vi "S8300E_voltage_test_WIH.vi"() -> ()   [LabVIEW 2011]
uses:
  Instance          16 28Saved   KT300WR2_TP125B_PCBA .vi
  Instance          20 28Saved   KT300WR2_TP125B_PCBA .vi
panel:
  out "history log":string
  out "Log1":string
  out "DDR3 HL":string
  out "VRH":string[](array[string])
  out "VRL":string[](array[string])
  out "Measure Ai name":string
  out "VISA resource name out":refnum<visa-resource-name>
  out "SEARCHING Test Item":string[](array[string])
  out "SFCS_Network Ok?":bool=TRUE
  out "log_measured Voltage":string
  out "begin time":u32
  out "All Pass?":bool=TRUE
  out "Result(測試總結果)":bool
  out "Total TP":i32
  out "record(s)":T1(array[cluster])
  out "狀況":string
  out "Test Result (測試結果)":T2(array[cluster])
  # "S8300E  Voltage Test Points Check"
  # "2015-6-1"
  # "COM9  Baud 115200"
  # "Error Code\nP5V\nP3V3\nP1V8\nPVCCIO\nP1V0_PCH\nPVCCSA\nH-P1V5\nH-P0V75\nPVCCPLL\nP3V3_S0\nP1V05_PCH\nP1V5_PCH\nP1V8_PCH\n P3V3_PCH\nL-P1V5\nL-P0V75"
types:
  T1 = cluster{"TestPoint_Name":string, "Lower Limit Voltage":dbl, "High Limit Voltage":dbl, cluster{"Relay3 Name":string, "Relay3H/L":bool}[], "Measure Ai name":string}[]
  T2 = cluster{"Test Item":string, "SPEC MIN ":dbl, "SPEC MAX ":dbl, "Measured":dbl, bool}[]
  T3 = enum16{"open", "replace", "create", "open or create", "replace or create", "replace or create with confirmation"}
  T4 = cluster{"Test Item":string, "SPEC MIN V":dbl, "SPEC MAX V":dbl, "Measured V":dbl, bool}[]
  T5 = cluster{"Test Item":string, "SPEC MIN C":dbl, "SPEC MAX C":dbl, "Measured C":dbl, bool}
  T6 = cluster{"Test Item":string, "SPEC MIN C":dbl, "SPEC MAX C":dbl, "Measured C":dbl, bool}[]
  T7 = cluster{"TestPoint_Name":string, "Lower Limit Voltage":dbl, "High Limit Voltage":dbl, cluster{"Relay3 Name":string, "Relay3H/L":bool}[], "Measure Ai name":string}
  T8 = cluster{"Relay3 Name":string, "Relay3H/L":bool}[]
  T9 = cluster{"Test Item":string, "SPEC MIN ":dbl, "SPEC MAX ":dbl, "Measured":dbl, bool}
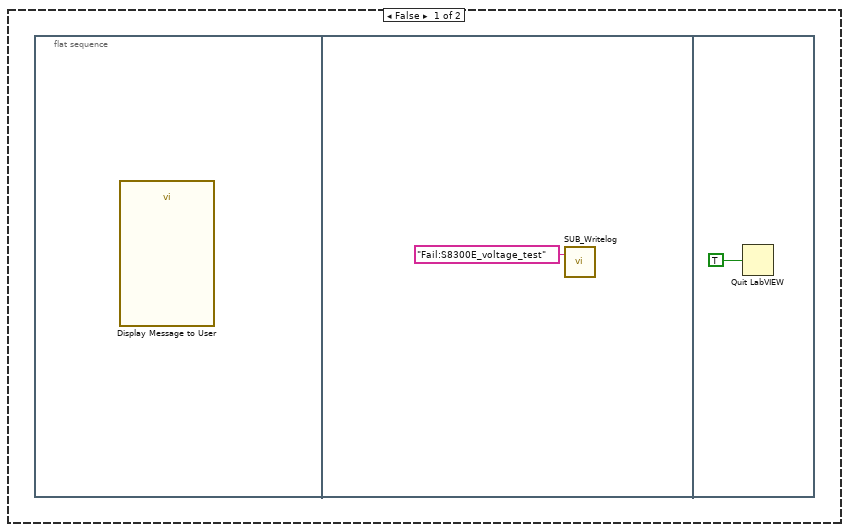
[diagram p2: hidden frame]
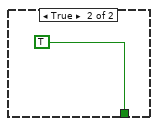
[diagram p5: hidden frame]
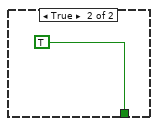
[diagram p8: hidden frame]
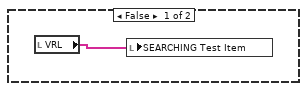
[diagram p9: hidden frame]
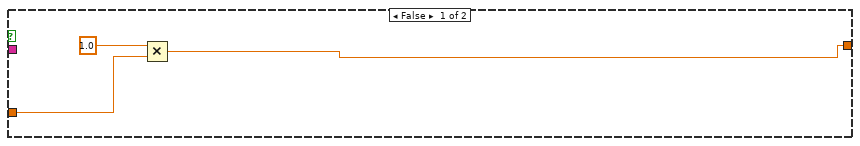
[diagram p12: hidden frame]
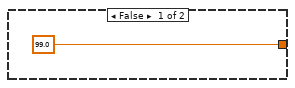
[diagram p13: hidden frame]
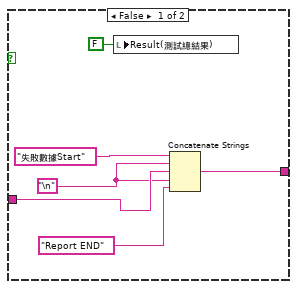
[diagram p15: hidden frame]
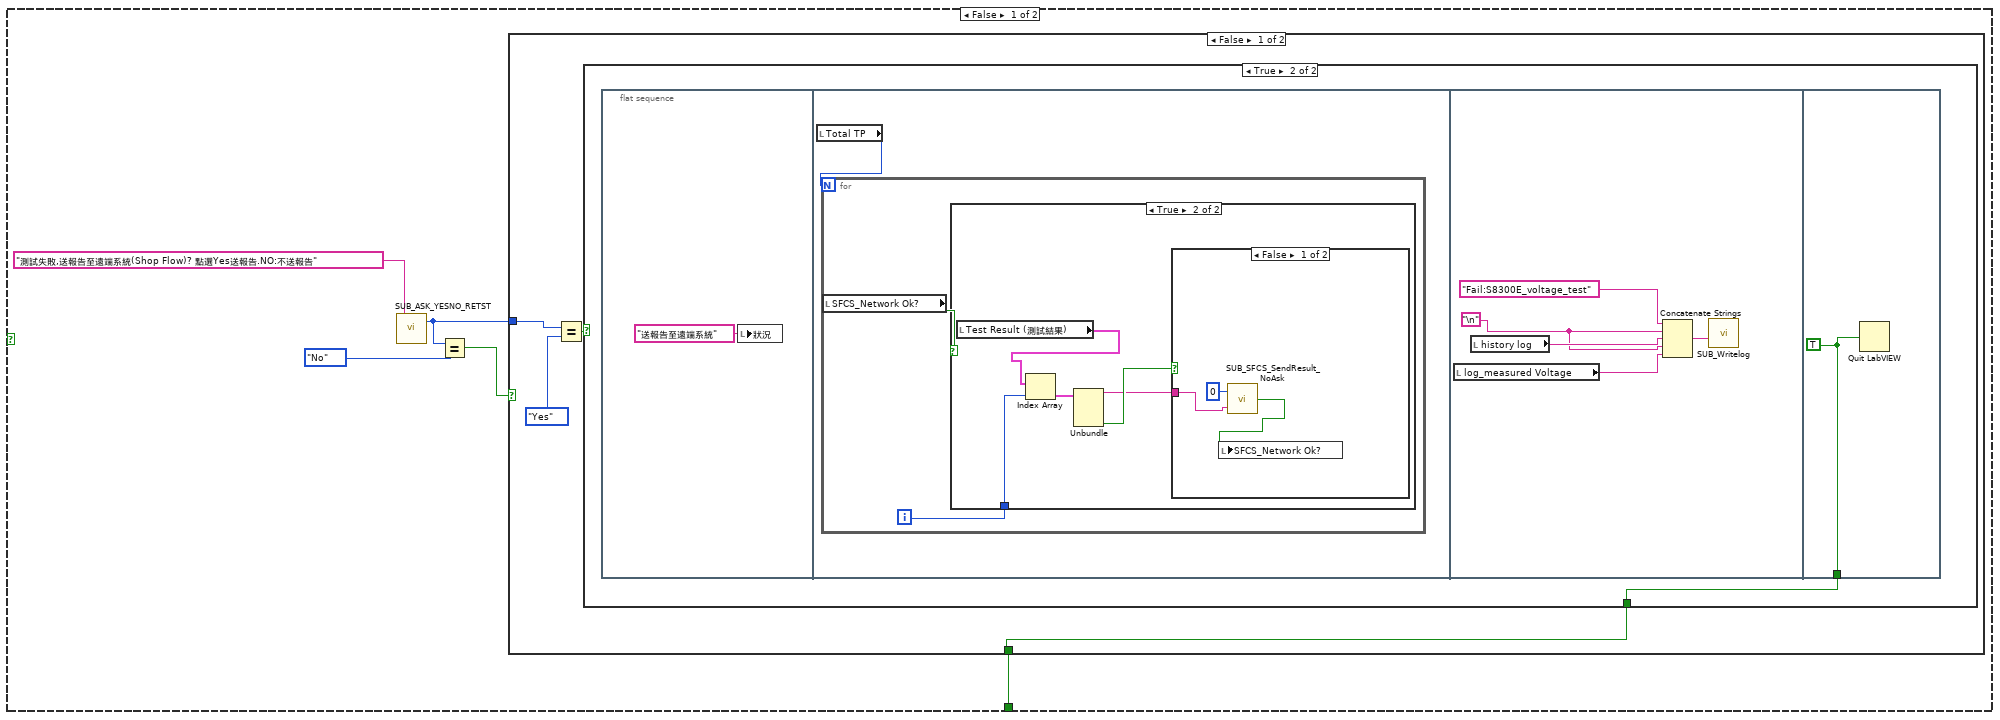
[diagram p16: hidden frame]
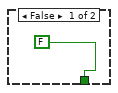
[diagram p17: hidden frame]
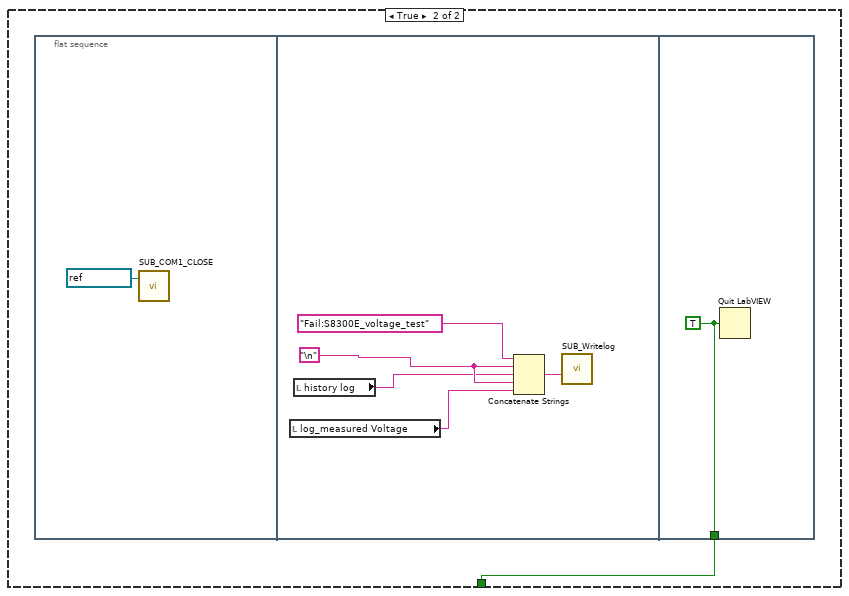
[diagram p20: hidden frame]
diagram:
  n1 = while {
    shift-right: [w4] -> _
    shift-left: "" -> [w3]
    stop <- w6 stop-if-true
    n2 = flat-sequence {
      tunnel: [w144] -> w5
      tunnel: w5 -> [w171]
      tunnel: [w270] -> w2
      tunnel: [w287] -> w6
      frame #0 {
        n3 = Tick Count (ms)() -> (millisecond timer value=→"begin time":u32)
      }
      frame #1 {
        n4 = property on="Result(測試總結果)" class="Bool (strict)"("Visible"=FALSE) -> ()  [unwired: 2 in, 2 out]
        n5 = property on="狀況" class="Str"("Blinking"=TRUE) -> ()  [unwired: 2 in, 2 out]
        "SFCS_Network Ok?" <- TRUE
        "狀況" <- ""
        "Result(測試總結果)" <- FALSE ("Result(測試總結果)")
        "All Pass?" <- TRUE
      }
      frame #2 {
        n6 = call "SUB_COM1_CLOSE.vi"("VISA resource name"=refnum<visa-resource-name> "COM9") -> ()  [unwired: 3 in]
      }
      frame #3 {
        n7 = call "SUB_COM9_INIT.vi"("baud rate"=u32 115200) -> ("VISA resource name out"=w15:refnum<visa-resource-name>)  [unwired: 1 in, 1 out]
        "VISA resource name out" <- w15
        n8 = call "SUB_ContinueCom1Read.vi"("Numeric"=1200, "duplicate VISA resource name 2"=w15) -> ()  [unwired: 1 in, 3 out]
      }
      frame #4 {
        n9 = call "SUB_SearchFile_inFolder.vi"("Search Filename in Folder"="S8300E_TP_Voltage.dat" ("name or relative path")) -> ("File Existing True/Flase"=w18:bool)  [unwired: 1 in]
        n10 = case shown="True" w18 {
          frame False {
            n11 = flat-sequence {
              frame #0 {
                n12 = call "Display Message to User"() -> ()  [unwired: 10 in, 2 out]
              }
              frame #1 {
                n13 = call "SUB_Writelog.vi"("Pass/Fail"="Fail:S8300E_voltage_test") -> ()  [unwired: 2 in]
              }
              frame #2 {
                n14 = Quit LabVIEW(quit? (T)=TRUE) -> ()
              }
            }
          }
          frame True {
            n15 = call "SUB_RunTime_FilePath.vi"() -> ("stripped path"=w24:path)  [unwired: 3 in]
            n16 = Build Path(base path=w24, name or relative path="S8300E_TP_Voltage.dat") -> (appended path=w31:path)
            n17 = Open/Create/Replace Datalog(5:T1 [] ("DatalogType"), 9:enum16{"read/write", "read-only", "write-only"}."read-only" ("access (0:read/write)"), 10:T3."open" ("operation (0:open)"), 11:w31) -> (0:w28:errorcluster, 3:w27:refnum<k1>)  [unwired: 2 in, 1 out]
            n18 = Read Datalog(4:w28, 7:w27) -> (0:w30:errorcluster, 2:w26:T1, 3:w29:refnum<k1>)  [unwired: 1 in]
            "record(s)" <- w26
            n19 = Array Size(array=w26) -> (size(s)=→"Total TP":i32)
            n20 = Close File(refnum=w29, error in=w30) -> ()  [unwired: 2 out]
          }
        }
      }
      frame #5 {
        n21 = case shown="True" TRUE {
          frame False {
          }
          frame True {
            n22 = while {
              stop <- w44 stop-if-true
              w36 = "S8300E" ("Find this String")
              w39 = "\r"
              n23 = local read "VISA resource name out"() -> (w40:refnum<visa-resource-name>)
              n24 = Concatenate Strings(w39, w39, w39) -> (w38:string)
              n25 = call "SUB_COM1Wrt.vi"("VISA resource name"=w40, "write buffer"=w38) -> ("duplicate VISA resource name"=w43:refnum<visa-resource-name>)  [unwired: 1 in, 1 out]
              n26 = Tick Count (ms)() -> (millisecond timer value=w42:u32)
              n27 = call "SUB_READ_COM1_FindString_timeout.vi"("Find this String"=w36, "Timeout Seccond"=5.0, "Begin time"=w42, "duplicate VISA resource name 2"=w43) -> ("Output String"=w35:string)  [unwired: 1 in, 2 out]
              n28 = call "SUB_FindSpecificString.vi"("Find this String"=w36, "String data"=w35) -> ("Found"=w37:bool)  [unwired: 2 in, 1 out]
              n29 = case shown="False" w37 {
                tunnel: w35 -> [w49 _]
                tunnel: [w45 TRUE] -> w44
                frame False {
                  n30 = call "SUB_YESNO.vi"("Debug View"=w49, "Status"="UART無正確反應!需有S8300E字串") -> ("yes/no"=w48:enum32{"No Selection", "Yes", "No", "None"})  [unwired: 1 in]
                  n31 = Equal?(x=w48, y=enum32{"No Selection", "Yes", "No", "None"}."No") -> (x = y?=w46:bool)
                  n32 = case shown="True" w46 {
                    tunnel: [_ w51] -> w45
                    frame False {
                    }
                    frame True {
                      n33 = flat-sequence {
                        tunnel: [w55] -> w51
                        frame #0 {
                          n34 = call "SUB_Writelog.vi"("Pass/Fail"="Fail:S8300E_voltage_test") -> ()  [unwired: 2 in]
                        }
                        frame #1 {
                          n35 = call "SUB_SFCS_SendResult.vi"("ErrorCode"="UART", "PASS_Fail (1/0)"=i8 0) -> ()  [unwired: 1 out]
                        }
                        frame #2 {
                          w55 = TRUE ("quit? (T)")
                          n36 = Quit LabVIEW(quit? (T)=w55) -> ()
                        }
                      }
                    }
                  }
                }
                frame True {
                }
              }
            }
          }
        }
      }
      frame #6 {
        # "這邊只是示範,如何從Records 找出欲測測點的\n資料"
        n37 = Build Array("P5V", "P3V3", "P1V8", "PVCCIO", "P1V0_PCH", "PVCCSA", "H-P1V5", "H-P0V75", "PVCCPLL", "P3V3_S0", "P1V05_PCH", "P1V5_PCH", "P1V8_PCH", "P3V3_PCH") -> (w57:string[])
        "VRH" <- w57
        n38 = Array Size(array=w57) -> (size(s)=w72:i32)
        n39 = local write "Total TP"(w72) -> ()
      }
      frame #7 {
        n40 = Build Array("P5V", "P3V3", "P1V8", "PVCCIO", "P1V0_PCH", "PVCCSA", "L-P1V5", "L-P0V75", "PVCCPLL", "P3V3_S0", "P1V05_PCH", "P1V5_PCH", "P1V8_PCH", "P3V3_PCH") -> (→"VRL":string[])
      }
      frame #8 {
        # "Dummy Command"
        n41 = local read "VISA resource name out"() -> (w92:refnum<visa-resource-name>)
        n42 = Concatenate Strings("./volt.sh 1" ("string"), "\r") -> (w93:string)
        n43 = call "SUB_COM1Wrt.vi"("VISA resource name"=w92, "write buffer"=w93) -> ("duplicate VISA resource name"=w88:refnum<visa-resource-name>)  [unwired: 1 in, 1 out]
        n44 = call "SUB_ContinueCom1Read.vi"("Numeric"=12000, "duplicate VISA resource name 2"=w88) -> ()  [unwired: 1 in, 3 out]
      }
      frame #9 {
        n45 = case shown="True" TRUE {
          frame False {
          }
          frame True {
            n46 = while {
              stop <- w113 stop-if-true
              n47 = local read "VISA resource name out"() -> (w101:refnum<visa-resource-name>)
              n48 = Tick Count (ms)() -> (millisecond timer value=w98:u32)
              n49 = Concatenate Strings("./mem.sh -v ", "\r") -> (w102:string)
              n50 = call "SUB_COM1Wrt.vi"("VISA resource name"=w101, "write buffer"=w102) -> ("duplicate VISA resource name"=w100:refnum<visa-resource-name>)  [unwired: 1 in, 1 out]
              n51 = call "SUB_COM_NoErrRead_TimeOut.vi"("Timeout Seccond"=5.0, "Begin time"=w98, "Find this String"="PASSED=", "VISA resource name"=w100) -> ("concatenated string"=w95:string, "Found"=w96:bool)  [unwired: 4 in]
              "Log1" <- w95
              n52 = call "SUB_FindSpecificString.vi"("Find this String"="PASSED=0x00", "String data"=w95) -> ("Found"=w107:bool)  [unwired: 2 in, 1 out]
              n53 = call "SUB_FindSpecificString.vi"("Find this String"="PASSED=", "String data"=w95) -> ("before \"; \" string"=→"DDR3 HL":string)  [unwired: 2 in, 1 out]
              n54 = call "SUB_FindSpecificString.vi"("Find this String"="PASSED=0x01", "String data"=w95) -> ("Found"=w106:bool)  [unwired: 2 in, 1 out]
              n55 = Or(x=w107, y=w106) -> (x .or. y?=w104:bool)
              n56 = And(x=w96, y=w104) -> (x .and. y?=w105:bool)
              n57 = case shown="False" w105 {
                tunnel: [w115 TRUE] -> w113
                tunnel: w95 -> [w114 _]
                frame False {
                  n58 = call "SUB_YESNO.vi"("Debug View"=w114, "Status"="UART無正確反應!需有PASSED=0x01或PASSED=0x00字串") -> ("yes/no"=w118:enum32{"No Selection", "Yes", "No", "None"})  [unwired: 1 in]
                  n59 = Equal?(x=w118, y=enum32{"No Selection", "Yes", "No", "None"}."No") -> (x = y?=w116:bool)
                  n60 = case shown="True" w116 {
                    tunnel: [_ w120] -> w115
                    frame False {
                    }
                    frame True {
                      n61 = flat-sequence {
                        tunnel: [w124] -> w120
                        frame #0 {
                          n62 = call "SUB_Writelog.vi"("Pass/Fail"="Fail:S8300E_voltage_test") -> ()  [unwired: 2 in]
                        }
                        frame #1 {
                          n63 = call "SUB_SFCS_SendResult.vi"("ErrorCode"="UART", "PASS_Fail (1/0)"=i8 0) -> ()  [unwired: 1 out]
                        }
                        frame #2 {
                          w124 = TRUE ("quit? (T)")
                          n64 = Quit LabVIEW(quit? (T)=w124) -> ()
                        }
                      }
                    }
                  }
                }
                frame True {
                }
              }
            }
          }
        }
      }
      frame #10 {
        "SEARCHING Test Item" <- string[] [] ("SEARCHING Test Item")
      }
      frame #11 {
        n65 = local read "DDR3 HL"() -> (w131:string)
        n66 = To Upper Case(1:w131) -> (0:w129:string)
        n67 = To Upper Case(1:"0x01" ("string")) -> (0:w128:string)
        n68 = Equal?(x=w129, y=w128) -> (x = y?=w127:bool)
        n69 = case shown="True" w127 {
          frame False {
            n70 = local read "VRL"() -> (w132:string[])
            n71 = local write "SEARCHING Test Item"(w132) -> ()
          }
          frame True {
            n72 = local read "VRH"() -> (w133:string[])
            n73 = local write "SEARCHING Test Item"(w133) -> ()
          }
        }
      }
      frame #12 {
        n74 = local read "Total TP"() -> (w136:i32)
        n75 = for {
          N: w136 -> [_]
          shift-right: [w139] -> w134
          shift-left: T4 [] -> [w137]
          n76 = call "SUB_TP_Output.vi"("Measured C"=-1.0 ("Measured V"), "SPEC MAX C"=0.0 ("SPEC MAX V"), "SPEC MIN C"=0.0 ("SPEC MIN V"), "Test Item"="") -> ("result"=w138:T5)  [unwired: 2 out]
          n77 = Build Array (concatenate)(w137, w138) -> (w139:T6)
        }
        "Test Result (測試結果)" <- w134
      }
      frame #13 {
        n78 = local read "Total TP"() -> (w146:i32)
        n79 = for {
          N: w146 -> [_]
          shift-right: [w148] -> w144
          shift-left: T1 [] -> [w147]
          i -> [w153]
          n80 = local read "SEARCHING Test Item"() -> (w154:string[])
          n81 = Index Array(array=w154, index=w153) -> (element=w151:string)
          n82 = call <vilib>:"Trim Whitespace.vi"("string"=w151) -> ("trimmed string"=w152:string)  [unwired: 1 in]
          n83 = To Upper Case(1:w152) -> (0:w150:string)
          n84 = while {
            tunnel: w150 -> [w160]
            tunnel: [w158] -> w149
            i -> [w155]
            stop <- w166 stop-if-true
            n85 = local read "record(s)"() -> (w164:T1)
            n86 = Array Size(array=w164) -> (size(s)=w156:i32)
            n87 = Index Array(array=w164, index=w155) -> (element=w157:T7)
            n88 = Unbundle By Name(w157) -> ("TestPoint_Name"=w163:string)
            n89 = call <vilib>:"Trim Whitespace.vi"("string"=w163) -> ("trimmed string"=w162:string)  [unwired: 1 in]
            n90 = To Upper Case(1:w162) -> (0:w161:string)
            n91 = Greater Or Equal?(x=w155, y=w156) -> (x >= y?=w165:bool)
            n92 = Equal?(x=w161, y=w160) -> (x = y?=w159:bool)
            n93 = case shown="True" w159 {
              tunnel: [_ w167] -> w158
              tunnel: w157 -> [_ w167]
              frame False {
              }
              frame True {
              }
            }
            n94 = Or(x=w159, y=w165) -> (x .or. y?=w166:bool)
          }
          n95 = Build Array (concatenate)(w147, w149) -> (w148:T1)
        }
        n96 = local write "record(s)"(w144) -> ()
      }
      frame #14 {
        n97 = local read "Total TP"() -> (w169:i32)
        n98 = Array Size(array=w171) -> (size(s)=w168:i32)
        n99 = Not Equal?(x=w168, y=w169) -> (x != y?=w170:bool)
        n100 = case shown="True" w170 {
          tunnel: w169 -> [_ w173]
          tunnel: w168 -> [_ w172]
          frame False {
          }
          frame True {
            n101 = flat-sequence {
              tunnel: w173 -> [w185]
              tunnel: w172 -> [w179]
              frame #0 {
                n102 = Number To Decimal String(number=w185) -> (decimal integer string=w183:string)  [unwired: 1 in]
                n103 = Number To Decimal String(number=w179) -> (decimal integer string=w178:string)  [unwired: 1 in]
                n104 = Concatenate Strings("失敗!", "需找", w183, "筆", "\r", "但實際上找找到", w178, "筆", "\r") -> (w175:string)
                n105 = call "Display Message to User3"("Message"=w175) -> ()  [unwired: 9 in, 2 out]
              }
              frame #1 {
                n106 = call "SUB_Writelog.vi"("Pass/Fail"="Fail:S8300E_voltage_test") -> ()  [unwired: 2 in]
              }
              frame #2 {
                n107 = Quit LabVIEW(quit? (T)=TRUE) -> ()
              }
            }
          }
        }
      }
      frame #15 {
        n108 = local read "Total TP"() -> (w190:i32)
        n109 = for {
          N: w190 -> [_]
          shift-right: [w203] -> w188
          shift-left: "" -> [w202]
          i -> [w194]
          n110 = flat-sequence {
            tunnel: w194 -> [w216]
            tunnel: [w212] -> w201
            tunnel: [w210] -> w200
            tunnel: [w211] -> w199
            tunnel: [w213] -> w198
            tunnel: [w204] -> w191
            tunnel: w194 -> [w235]
            tunnel: w201 -> [w222]
            tunnel: w200 -> [w233]
            tunnel: w199 -> [w232]
            tunnel: [w227] -> w203
            tunnel: w202 -> [w226]
            tunnel: w198 -> [w224]
            tunnel: w191 -> [w218]
            frame #0 {
              n111 = local read "record(s)"() -> (w217:T1)
              n112 = Index Array(array=w217, index=w216) -> (element=w209:T7)
              n113 = Unbundle By Name(w209) -> ("TestPoint_Name"=w212:string, "Lower Limit Voltage"=w210:dbl, "High Limit Voltage"=w211:dbl, "Measure Ai name"=w213:string)
              n114 = Unbundle(w209) -> (w208:T8)  [unwired: 4 out]
              n115 = Index Array(array=w208, index=0) -> (element=w206:cluster{"Relay3 Name":string, "Relay3H/L":bool})
              n116 = Concatenate Strings(w212, "  測點測試中..." ("string")) -> (w215:string)
              n117 = Unbundle(w206) -> ("Relay3 Name"=w205:string)  [unwired: 1 out]
              n118 = local write "狀況"(w215) -> ()
              n119 = Fract/Exp String To Number(string=w205) -> (number=w204:dbl)  [unwired: 3 in, 1 out]
            }
            frame #1 {
              n120 = case shown="True" TRUE {
                tunnel: [w237 w248] -> w225
                tunnel: w224 -> [_ w250]
                tunnel: w218 -> [w238 w240]
                frame False {
                  n121 = Multiply(x=1.0 ("AVG_Vol"), y=w238) -> (x*y=w237:dbl)
                }
                frame True {
                  w241 = "PASSED=" ("Find this String")
                  n122 = local read "VISA resource name out"() -> (w252:refnum<visa-resource-name>)
                  n123 = Concatenate Strings(w250, "\r") -> (w249:string)
                  n124 = call "SUB_COM1Wrt.vi"("VISA resource name"=w252, "write buffer"=w249) -> ("duplicate VISA resource name"=w247:refnum<visa-resource-name>)  [unwired: 1 in, 1 out]
                  n125 = Tick Count (ms)() -> (millisecond timer value=w246:u32)
                  n126 = call "SUB_READ_COM1_FindString_timeout.vi"("Find this String"=w241, "Timeout Seccond"=2.0, "Begin time"=w246, "duplicate VISA resource name 2"=w247) -> ("Output String"=w242:string, "Found String"=w244:bool)  [unwired: 1 in, 1 out]
                  n127 = call "SUB_FindSpecificString.vi"("Find this String"=w241, "String data"=w242) -> ("before \"; \" string"=w243:string)  [unwired: 2 in, 1 out]
                  n128 = case shown="True" w244 {
                    tunnel: w243 -> [_ w263]
                    tunnel: [99.0 w256] -> w248
                    tunnel: w240 -> [_ w254]
                    frame False {
                    }
                    frame True {
                      w258 = "簞"
                      n129 = call "SUB_OUT_THIS_token.vi"("Remove token symbl1 3"="C", "Remove token symbl1 2"="~", "Remove token symbl1"="+", "input string"=w263) -> ("result string"=w259:string)  [unwired: 1 in]
                      n130 = call "SUB_OUT_THIS_token.vi"("Remove token symbl1 3"=w258, "Remove token symbl1 2"=w258, "Remove token symbl1"=w258, "input string"=w259) -> ("result string"=w257:string)  [unwired: 1 in]
                      n131 = Fract/Exp String To Number(string=w257) -> (number=w255:dbl)  [unwired: 3 in, 1 out]
                      n132 = Multiply(x=w255, y=w254) -> (x*y=w256:dbl)
                    }
                  }
                }
              }
              n133 = local read "Test Result (測試結果)"() -> (w236:T2)
              n134 = call "SUB_TP_Output.vi"("Measured C"=w225, "SPEC MAX C"=w232, "SPEC MIN C"=w233, "Test Item"=w222) -> ("result"=w231:T5)  [unwired: 2 out]
              n135 = Number To Fractional String(number=w225, precision (6)=i16 2) -> (F-format string=w229:string)  [unwired: 2 in]
              n136 = Replace Array Subset(array=w236, new element=w231, index=w235) -> (w234:T2)
              n137 = local write "Test Result (測試結果)"(w234) -> ()
              n138 = Concatenate Strings(w222, "=" ("string"), w229, ";", "\n") -> (w228:string)
              n139 = Concatenate Strings(w226, w228) -> (w227:string)
              "Measure Ai name" <- w224
            }
          }
          n140 = Subtract(x=w194, y=5) -> (x-y=w197:i32)
          n141 = In Range and Coerce(upper limit=w194, x=w197, lower limit=0.0) -> (coerced(x)=w193:dbl)  [unwired: 1 out]
          n142 = Build Array(w193) -> (w192:dbl[])
          n143 = property on="Test Result (測試結果)" class="Arr (strict)"("Index Values"=w192) -> ()  [unwired: 2 in, 2 out]
        }
        "log_measured Voltage" <- w188
      }
      frame #16 {
        n144 = local read "Total TP"() -> (w264:i32)
        n145 = for {
          N: w264 -> [_]
          i -> [w267]
          n146 = local read "Test Result (測試結果)"() -> (w268:T2)
          n147 = Index Array(array=w268, index=w267) -> (element=w266:T9)
          n148 = Unbundle(w266) -> (w265:bool)  [unwired: 4 out]
          n149 = case shown="False" w265 {
            frame False {
              n150 = local write "All Pass?"(FALSE ("All Pass?")) -> ()
            }
            frame True {
            }
          }
        }
      }
      frame #17 {
        n151 = local read "log_measured Voltage"() -> (w271:string)
        n152 = local read "All Pass?"() -> (w272:bool)
        n153 = case shown="True" w272 {
          tunnel: w271 -> [w276 w280]
          tunnel: [w273 w279] -> w270
          frame False {
            w275 = "\n"
            n154 = local write "Result(測試總結果)"(FALSE ("Result(測試總結果)")) -> ()
            n155 = Concatenate Strings("失敗數據Start" ("string"), w275, w276, w275, "Report END" ("string")) -> (w273:string)
          }
          frame True {
            w282 = "\n"
            n156 = local write "Result(測試總結果)"(TRUE ("Result(測試總結果)")) -> ()
            n157 = Concatenate Strings("成功數據Start" ("string"), w282, w280, w282, "Report END" ("string")) -> (w279:string)
          }
        }
      }
      frame #18 {
        n158 = local write "SFCS_Network Ok?"(TRUE ("SFCS_Network Ok?")) -> ()
        n159 = property on="Result(測試總結果)" class="Bool (strict)"("Visible"=TRUE) -> ()  [unwired: 2 in, 2 out]
      }
      frame #19 {
        n160 = local read "All Pass?"() -> (w288:bool)
        n161 = case shown="True" w288 {
          tunnel: [w290 w326] -> w287
          frame False {
            n162 = call "SUB_ASK_YESNO_RETST.vi"("Question:"="測試失敗,送報告至遠端系統(Shop Flow)? 點選Yes送報告.NO:不送報告") -> ("yes/no"=w289:enum32{"No Selection", "Yes", "No", "None"})  [unwired: 2 in]
            n163 = Equal?(x=w289, y=enum32{"No Selection", "Yes", "No", "None"}."No") -> (x = y?=w291:bool)
            n164 = case shown="False" w291 {
              tunnel: [w297 w318] -> w290
              tunnel: w289 -> [w295 _]
              frame False {
                n165 = Equal?(x=w295, y=enum32{"No Selection", "Yes", "No", "None"}."Yes") -> (x = y?=w296:bool)
                n166 = case shown="True" w296 {
                  tunnel: [FALSE w299] -> w297
                  frame False {
                  }
                  frame True {
                    n167 = flat-sequence {
                      tunnel: [w317] -> w299
                      frame #0 {
                        n168 = local write "狀況"("送報告至遠端系統" ("狀況")) -> ()
                      }
                      frame #1 {
                        n169 = local read "Total TP"() -> (w301:i32)
                        n170 = for {
                          N: w301 -> [_]
                          i -> [w303]
                          n171 = local read "SFCS_Network Ok?"() -> (w302:bool)
                          n172 = case shown="True" w302 {
                            tunnel: w303 -> [_ w307]
                            frame False {
                            }
                            frame True {
                              n173 = local read "Test Result (測試結果)"() -> (w308:T2)
                              n174 = Index Array(array=w308, index=w307) -> (element=w306:T9)
                              n175 = Unbundle(w306) -> ("Test Item"=w304:string, w305:bool)  [unwired: 3 out]
                              n176 = case shown="False" w305 {
                                tunnel: w304 -> [w310 _]
                                frame False {
                                n177 = call "SUB_SFCS_SendResult_NoAsk.vi"("ErrorCode"=w310, "PASS_Fail (1/0)"=i8 0) -> ("Sent OK ?"=w309:bool)
                                n178 = local write "SFCS_Network Ok?"(w309) -> ()
                                }
                                frame True {
                                }
                              }
                            }
                          }
                        }
                      }
                      frame #2 {
                        w313 = "\n"
                        n179 = local read "log_measured Voltage"() -> (w312:string)
                        n180 = local read "history log"() -> (w314:string)
                        n181 = Concatenate Strings("Fail:S8300E_voltage_test", w313, w314, w313, w312) -> (w316:string)
                        n182 = call "SUB_Writelog.vi"("Pass/Fail"=w316) -> ()  [unwired: 2 in]
                      }
                      frame #3 {
                        w317 = TRUE ("quit? (T)")
                        n183 = Quit LabVIEW(quit? (T)=w317) -> ()
                      }
                    }
                  }
                }
              }
              frame True {
                n184 = flat-sequence {
                  tunnel: [w325] -> w318
                  frame #0 {
                    n185 = call "SUB_COM1_CLOSE.vi"("VISA resource name"=refnum<visa-resource-name> "COM9") -> ()  [unwired: 3 in]
                  }
                  frame #1 {
                    w322 = "\n"
                    n186 = local read "log_measured Voltage"() -> (w320:string)
                    n187 = local read "history log"() -> (w321:string)
                    n188 = Concatenate Strings("Fail:S8300E_voltage_test", w322, w321, w322, w320) -> (w324:string)
                    n189 = call "SUB_Writelog.vi"("Pass/Fail"=w324) -> ()  [unwired: 2 in]
                  }
                  frame #2 {
                    w325 = TRUE ("quit? (T)")
                    n190 = Quit LabVIEW(quit? (T)=w325) -> ()
                  }
                }
              }
            }
          }
          frame True {
            n191 = flat-sequence {
              tunnel: [TRUE] -> w326
              frame #0 {
                n192 = case shown="True" TRUE {
                  frame False {
                  }
                  frame True {
                    n193 = call "SUB_COM1_CLOSE.vi"("VISA resource name"=refnum<visa-resource-name> "COM9") -> ()  [unwired: 3 in]
                  }
                }
              }
              frame #1 {
                w331 = "***Not Good ***" ("replace string (\"\")")
                w336 = "\n"
                n194 = local read "history log"() -> (w335:string)
                n195 = local read "Log1"() -> (w337:string)
                n196 = local read "begin time"() -> (w342:u32)
                n197 = Tick Count (ms)() -> (millisecond timer value=w341:u32)
                n198 = call "SUB_CAL_TESTTIME.vi"("Test Item name"="S8300E_voltage_test", "Stop tick time"=w341, "Start tick time"=w342) -> ("Test Time output"=w338:string)  [unwired: 2 in]
                n199 = Concatenate Strings("Pass:S8300E_voltage_test", w336, w337, w336, w335, w338) -> (w330:string)
                n200 = call "SUB_SEARCH_REPLACE_STR.vi"("replace string (\"\")"=w331, "search string"="FAILED", "input string"=w330) -> ("result string"=w333:string)  [unwired: 2 in]
                n201 = call "SUB_SEARCH_REPLACE_STR.vi"("replace string (\"\")"=w331, "search string"="FAIL", "input string"=w333) -> ("result string"=w329:string)  [unwired: 2 in]
                n202 = call "SUB_Writelog.vi"("Pass/Fail"=w329) -> ()  [unwired: 2 in]
              }
              frame #2 {
                n203 = call "SUB_COM1_CLOSE.vi"("VISA resource name"=refnum<visa-resource-name> "COM9") -> ()  [unwired: 3 in]
              }
              frame #3 {
              }
              frame #4 {
                n204 = Quit LabVIEW(quit? (T)=TRUE) -> ()
              }
            }
          }
        }
      }
    }
    n205 = Concatenate Strings(w3, w2) -> (w4:string)
    "history log" <- w4
  }
